vi "PopulateRings.vi"(8 "error in (no error)":errorcluster, 11 "MAUI in":refnum<class "MAUI.lvclass">) -> (0 "error out":errorcluster, 3 "MAUI out":refnum<class "MAUI.lvclass">)   [LabVIEW 2019, in "MAUI.lvclass"]
uses:
  MAUI.lvclass
  MAUI.lvclass/MAUI.ctl
  <userlib>/LevyLab/Embedded UI/SMO.UI.Embedded/Embedded UI.lvclass
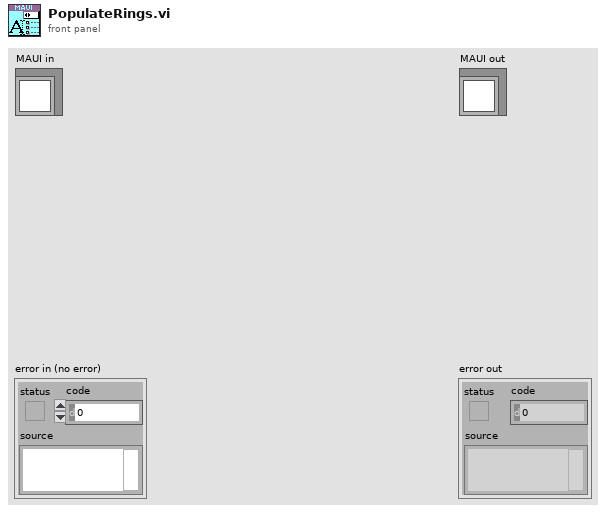
[diagram p1: front panel]
types:
  T1 = typedef "MAUI.lvclass/PanelData.ctl" = cluster{"SubPanel":refnum<vi>, "Ring":refnum<vi>, "Active":i32}
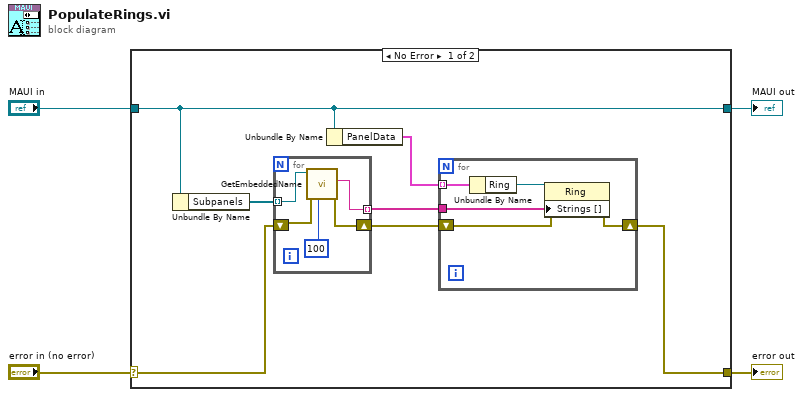
[diagram p0: block diagram]
diagram:
  n1 = case shown="No Error" "error in (no error)" {
    selector: "error in (no error)" -> [w11 w23]
    tunnel: [w9 w23] -> w3
    tunnel: [w8 w22] -> w1
    tunnel: "MAUI in" -> [w8 w22]
    frame No Error {
      n2 = Unbundle By Name(w8) -> ("Subpanels"=w7:refnum<class "Embedded UI.lvclass">[])
      n3 = for {
        tunnel: w7 -> [w19] mode=indexing
        tunnel: [w18] -> w5 mode=indexing
        shift-right: [w21] -> w10
        shift-left: w11 -> [w20]
        n4 = call <userlib>:"GetEmbeddedName.vi"("timeout in ms (-1)"=100, "error in (no error)"=w20, "EmbeddedSMO in"=w19) -> ("error out"=w21:errorcluster, "Name"=w18:string)  [unwired: 6 in, 1 out]
      }
      n5 = Unbundle By Name(w8) -> ("PanelData"=w6:T1[])
      n6 = for {
        tunnel: w6 -> [w14] mode=indexing
        tunnel: w5 -> [w12]
        shift-right: [w15] -> w9
        shift-left: w10 -> [w16]
        n7 = Unbundle By Name(w14) -> ("Ring"=w13:refnum<vi>)
        n8 = property class="Ring"(reference=w13, error in=w16, "Strings []"=w12) -> (error out=w15:errorcluster)  [unwired: 1 out]
      }
    }
    frame Error {
    }
  }
  "error out" <- w3
  "MAUI out" <- w1
